vi "average_with_for_loop.vi"() -> ()   [LabVIEW 2019]
panel:
  out "result":dbl
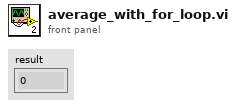
[diagram p1: front panel]
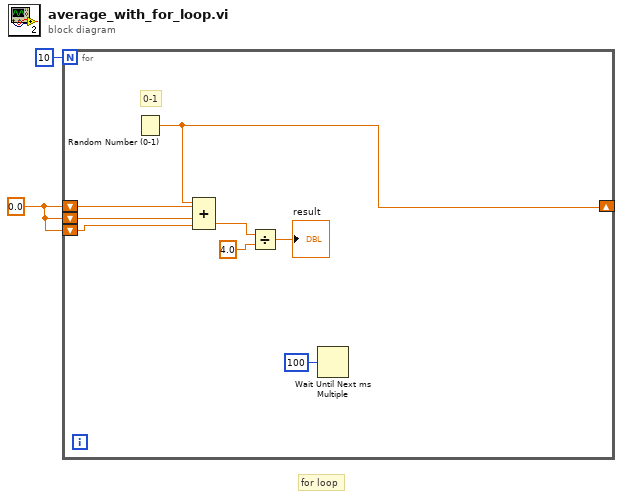
[diagram p0: block diagram]
diagram:
  w1 = 0.0 ("number: 0 to 1")
  # "for loop"
  n1 = for {
    N: 10 -> [_]
    shift-right: [w7] -> _
    shift-left: w1 -> [w6]
    shift-left: w1 -> [w5]
    shift-left: w1 -> [w4]
    # "0-1"
    n2 = Random Number (0-1)() -> (number: 0 to 1=w7:dbl)
    n3 = Compound Arithmetic op=ADD(w7, w6, w5, w4) -> (w9:dbl)
    n4 = Divide(x=w9, y=4.0) -> (x/y=→"result":dbl)
    n5 = Wait Until Next ms Multiple(millisecond multiple=u32 100) -> ()  [unwired: 1 out]
  }
